vi "Com_SECS Equipment _Control Message(Separate).vi"(8 "error in":errorcluster, 10 "Timeout":i32=1000, 11 "Buffer Data In":T1) -> (0 "error out":errorcluster, 3 "Buffer Data Out":T1)   [LabVIEW 2016]
uses:
  Data Def/Com_SECS Equipment _Buffer Data.ctl
  Data Def/Com_SECS Equipment _Connection Setting.ctl
  Data Def/Com_SECS Equipment _Timeout Setting.ctl
  Data Def/Com_SECS Equipment _SECS Packet.ctl
  Data Def/Com_SECS Equipment _Message Type.ctl
  Data Def/Com_SECS Equipment _Protocol Type.ctl
  Data Def/Com_SECS Equipment _Stream Type.ctl
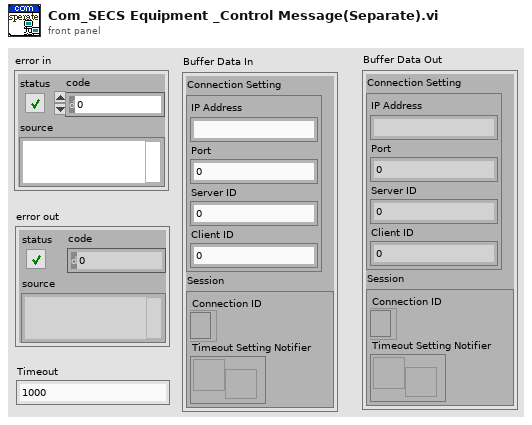
[diagram p1: front panel]
types:
  T1 = typedef "Com_SECS Equipment _Buffer Data.ctl" = cluster{"Connection Setting":T2, "Session":cluster{"Connection ID":refnum<k5>, "Timeout Setting Notifier":refnum<notifier>}}
  T2 = typedef "Com_SECS Equipment _Connection Setting.ctl" = cluster{"IP Address":string, "Port":u16, "Server ID":u16, "Client ID":u16}
  T3 = typedef "Com_SECS Equipment _Stream Type.ctl" = enum16{"Data Message", "Select.req", "Select.rsp", "Deselect.req", "Deselect.rsp", "Linktest.req", "Linktest.rsp", "Reject.req", "Separate.req", "Reserve"}
  T4 = typedef "Com_SECS Equipment _SECS Packet.ctl" = cluster{"Need Response?":bool, "Device ID":u16, "Stream":u8, "Function":u8, "Message Type":T5, "Protocol Type":T6, "Stream Type":T3, "System Btyes":u8[], "Message Data":u8[]}
  T5 = typedef "Com_SECS Equipment _Message Type.ctl" = enum16{"Control Message", "Data Message"}
  T6 = typedef "Com_SECS Equipment _Protocol Type.ctl" = enum16{"SECS-II Encoding", "Reserved"}
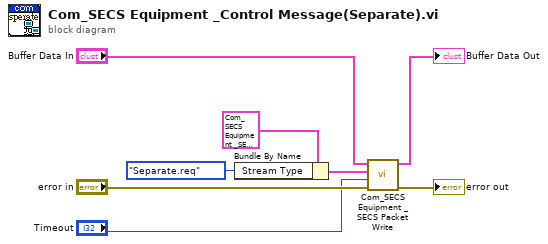
[diagram p0: block diagram]
diagram:
  n1 = Bundle By Name(cluster=T4 {"Need Response?"=FALSE, "Device ID"=0, "Stream"=0, "Function"=0, "Message Type"=enum."Control Message", "Protocol Type"=enum."SECS-II Encoding", "Stream Type"=enum."Linktest.req", "System Btyes"=[], "Message Data"=[]} ("SECS Packet"), "Stream Type"=Com_SECS_Equipment__Stream_Type."Separate.req") -> (w6:T4)
  n2 = call "Com_SECS Equipment _SECS Packet Write.vi"("error in"="error in", "Timeout"="Timeout", "SECS Packet"=w6, "Buffer Data In"="Buffer Data In") -> ("error out"=→"error out":errorcluster, "Buffer Data Out"=→"Buffer Data Out":T1)  [unwired: 6 in]
